vi "ReadVoltage_Core.vi"(6 "error in (no error)":errorcluster, 8 "Core PLL Instance":string(combo)="Core0", 9 "Voltage to Measure":string(combo)="Bandgap") -> (0 "error out":errorcluster, 3 "Voltage Read":dbl)   [LabVIEW 2011]
doc: "This VI reads a chosen voltage of a Core PLL instance.\n\nInputs:\n1. Voltage to Measure: Selects the voltage that will be read by the SRP ADC (ie. BG, VA, VD, etc.).\n2. Core PLL Instance: Selects the Core PLL instance to measure the voltage from (Core0, Core1, etc.).\n\nOutputs:\n1.Voltage Read: The value of the chosen measurement in volts."
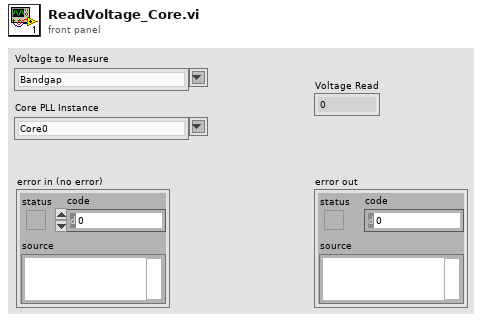
[diagram p1: front panel]
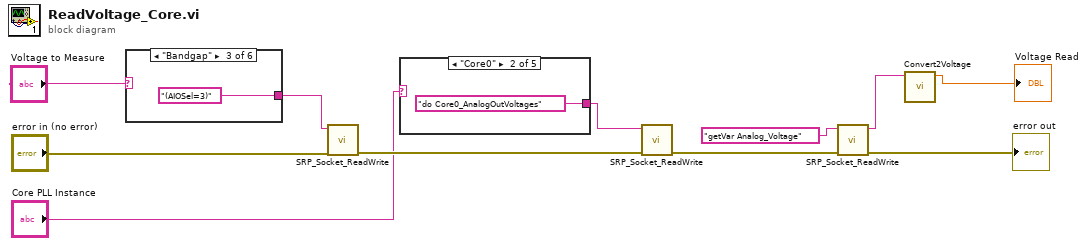
[diagram p0: block diagram]
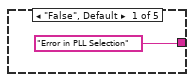
[diagram p2: hidden frame]
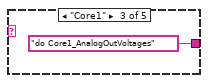
[diagram p3: hidden frame]
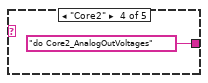
[diagram p4: hidden frame]
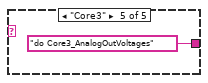
[diagram p5: hidden frame]
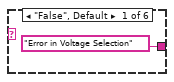
[diagram p6: hidden frame]
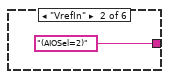
[diagram p7: hidden frame]
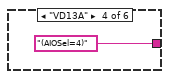
[diagram p8: hidden frame]
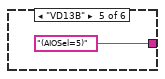
[diagram p9: hidden frame]
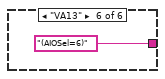
[diagram p10: hidden frame]
diagram:
  n1 = case shown="\"Bandgap\"" "Voltage to Measure" {
    tunnel: ["Error in Voltage Selection" "(AIOSel=2)" "(AIOSel=3)" "(AIOSel=4)" "(AIOSel=5)" "(AIOSel=6)"] -> w6
    frame "False", Default {
    }
    frame "VrefIn" {
    }
    frame "Bandgap" {
    }
    frame "VD13A" {
    }
    frame "VD13B" {
    }
    frame "VA13" {
    }
  }
  n2 = call "SRP_Socket_ReadWrite.vi"("error in (no error)"="error in (no error)", "Data In"=w6) -> ("error out"=w8:errorcluster)  [unwired: 7 in, 1 out]
  n3 = case shown="\"Core0\"" "Core PLL Instance" {
    tunnel: ["Error in PLL Selection" "do Core0_AnalogOutVoltages" "do Core1_AnalogOutVoltages" "do Core2_AnalogOutVoltages" "do Core3_AnalogOutVoltages"] -> w5
    frame "False", Default {
    }
    frame "Core0" {
    }
    frame "Core1" {
    }
    frame "Core2" {
    }
    frame "Core3" {
    }
  }
  n4 = call "SRP_Socket_ReadWrite.vi"("error in (no error)"=w8, "Data In"=w5) -> ("error out"=w9:errorcluster)  [unwired: 7 in, 1 out]
  n5 = call "SRP_Socket_ReadWrite.vi"("error in (no error)"=w9, "Data In"="getVar Analog_Voltage") -> ("error out"=→"error out":errorcluster, "Data Out"=w3:string)  [unwired: 7 in]
  n6 = call "Convert2Voltage.vi"("SRP ADC String"=w3) -> ("Voltage"=→"Voltage Read":dbl)  [unwired: 10 in]
